vi "Get Param Path & Name.vi"(11 "Path":string) -> (0 "Last Part":string, 1 "Parameter Path":string, 2 "Controller name":string)   [LabVIEW 2011]
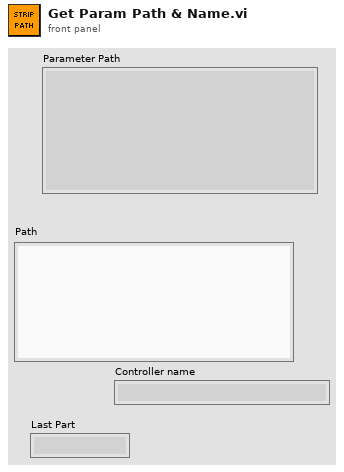
[diagram p1: front panel]
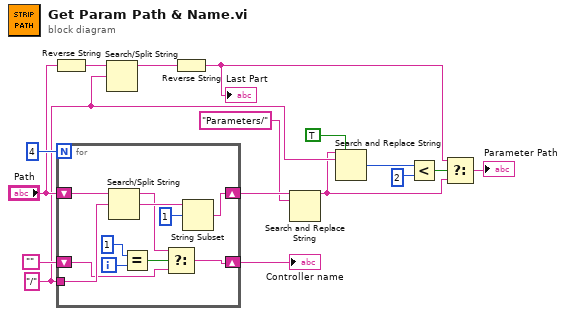
[diagram p0: block diagram]
diagram:
  w7 = "/" ("search string/char (-)")
  n1 = Reverse String(1:"Path") -> (0:w16:string)
  n2 = for {
    N: 4 -> [_]
    shift-right: [w24] -> w12
    shift-left: "Path" -> [w27]
    tunnel: w7 -> [w26]
    shift-right: [w18] -> w9
    shift-left: "" -> [w19]
    i -> [w22]
    n3 = Search/Split String(string=w27, search string/char (-)=w26) -> (substring before match=w17:string, match + rest of string=w25:string)  [unwired: 1 in, 1 out]
    n4 = Equal?(x=1, y=w22) -> (x = y?=w20:bool)
    n5 = Select(t=w17, s=w20, f=w19) -> (s? t:f=w18:string)
    n6 = String Subset(string=w25, offset (0)=1) -> (substring=w24:string)  [unwired: 1 in]
  }
  "Controller name" <- w9
  n7 = Search/Split String(string=w16, search string/char (-)=w7) -> (substring before match=w15:string)  [unwired: 1 in, 2 out]
  n8 = Reverse String(1:w15) -> (0:w3:string)
  "Last Part" <- w3
  n9 = Search and Replace String(input string=w12, search string="Parameters/") -> (result string=w2:string)  [unwired: 6 in, 3 out]
  n10 = Search and Replace String(replace all?=TRUE ("replace all? (F)"), input string=w2, search string=w7) -> (number of replacements=w6:i32)  [unwired: 5 in, 3 out]
  n11 = Less?(x=w6, y=2) -> (x < y?=w4:bool)
  n12 = Select(t=w3, s=w4, f=w2) -> (s? t:f=→"Parameter Path":string)
